vi "Analyte Molecule.vi"(4 "m-nm Gap Molecules":dbl caption="m-nm Gap", 6 "Gap Between Molecules":dbl caption="Gap Between CNTs", 7 "Radius of Molecule":dbl caption="Radius of CNTs", 9 "m-nm l Molecule":dbl, 10 "Length of Molecule":dbl caption="Length of CNTs", 11 "m-nm r Molecule":dbl caption="m-nm r") -> (1 "Molecule Length":dbl, 2 "Volume of Molecule":dbl, 3 "Molecle Area with Gap":dbl, 5 "Area of Molecule on CNT surface":dbl)   [LabVIEW 2020]
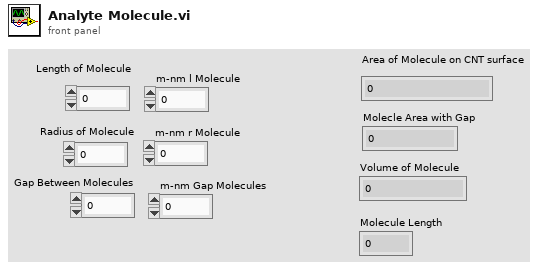
[diagram p1: front panel]
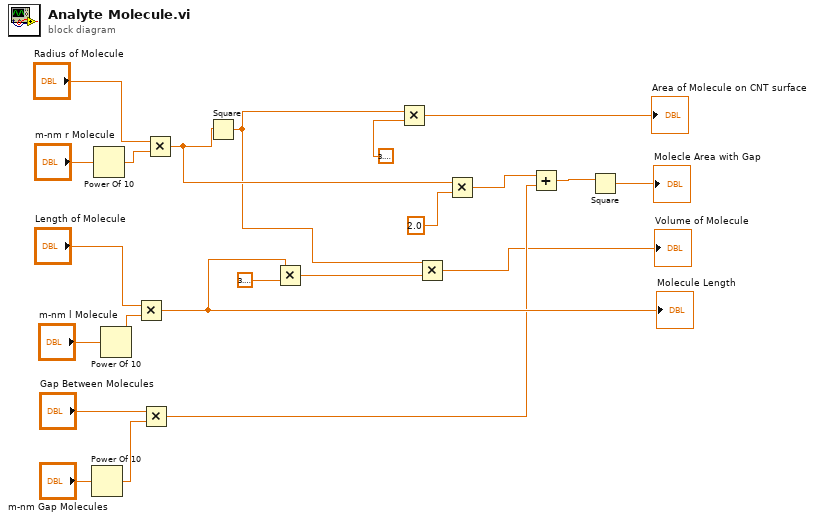
[diagram p0: block diagram]
diagram:
  n1 = Power Of 10(x="m-nm Gap Molecules") -> (10^x=w8:dbl)
  n2 = Power Of 10(x="m-nm r Molecule") -> (10^x=w2:dbl)
  n3 = Power Of 10(x="m-nm l Molecule") -> (10^x=w4:dbl)
  n4 = Multiply(x="Length of Molecule", y=w4) -> (x*y=w22:dbl)
  "Molecule Length" <- w22
  n5 = Multiply(x="Gap Between Molecules", y=w8) -> (x*y=w18:dbl)
  n6 = Multiply(x="Radius of Molecule", y=w2) -> (x*y=w21:dbl)
  n7 = Square(x=w21) -> (x^2=w20:dbl)
  n8 = Multiply(x=w22, y=3.141592653589793) -> (x*y=w13:dbl)
  n9 = Multiply(x=w20, y=3.141592653589793) -> (x*y=→"Area of Molecule on CNT surface":dbl)
  n10 = Multiply(x=w20, y=w13) -> (x*y=→"Volume of Molecule":dbl)
  n11 = Multiply(x=w21, y=2.0) -> (x*y=w19:dbl)
  n12 = Add(x=w19, y=w18) -> (x+y=w17:dbl)
  n13 = Square(x=w17) -> (x^2=→"Molecle Area with Gap":dbl)
